vi "Begin Scripting Session.vi"(8 "error in":errorcluster, 10 "Undo Name":string, 11 "VI in":refnum<vi>) -> (0 "error out":errorcluster, 2 "Scripting Session":T1, 3 "VI out":refnum<vi>)   [LabVIEW 2020, in "Enclose in Structure.lvlib"]
uses:
  Enclose in Structure.lvlib
  Scripting Session.ctl
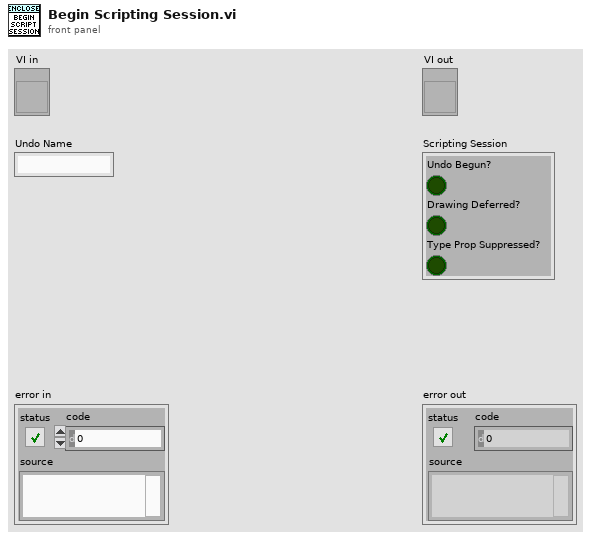
[diagram p1: front panel]
types:
  T1 = typedef "Enclose in Structure.lvlib/Scripting Session.ctl" = cluster{"Undo Begun?":bool, "Drawing Deferred?":bool, "Type Prop Suppressed?":bool}
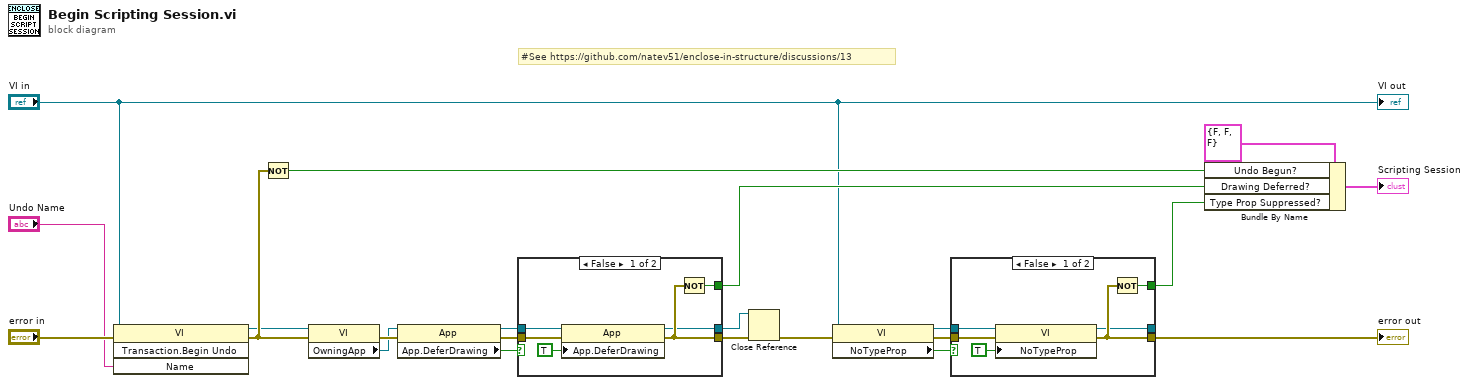
[diagram p0: block diagram]
diagram:
  # "#See https://github.com/natev51/enclose-in-structure/discussions/13"
  n1 = invoke class="VI" method="Transaction.Begin Undo"(reference="VI in", error in="error in", "Name"="Undo Name") -> (reference out=w4:refnum<vi>, error out=w22:errorcluster)  [unwired: 1 in, 2 out]
  n2 = Not(x=w22) -> (.not. x?=w2:bool)
  n3 = property class="VI"(reference=w4, error in=w22) -> (error out=w20:errorcluster, "OwningApp"=w19:refnum<vi>)  [unwired: 1 out]
  n4 = property class="App"(reference=w19, error in=w20) -> (reference out=w17:refnum<vi>, error out=w21:errorcluster, "App.DeferDrawing"=w13:bool)
  n5 = case shown="False" w13 {
    tunnel: w21 -> [w27 w29]
    tunnel: w17 -> [w26 w30]
    tunnel: [w28 w29] -> w16
    tunnel: [w25 w30] -> w15
    tunnel: [w23 _] -> w14
    frame False {
      n6 = property class="App"(reference=w26, error in=w27, "App.DeferDrawing"=TRUE ("Application:Defer Drawing")) -> (reference out=w25:refnum<vi>, error out=w28:errorcluster)
      n7 = Not(x=w28) -> (.not. x?=w23:bool)
    }
    frame True {
    }
  }
  n8 = Close Reference(reference=w15, error in (no error)=w16) -> (error out=w9:errorcluster)
  n9 = property class="VI"(reference="VI in", error in=w9) -> (reference out=w11:refnum<vi>, error out=w10:errorcluster, "NoTypeProp"=w12:bool)
  n10 = case shown="False" w12 {
    tunnel: w10 -> [w35 w37]
    tunnel: w11 -> [w34 w38]
    tunnel: [w36 w37] -> w6
    tunnel: [w33 w38] -> _
    tunnel: [w32 _] -> w8
    frame False {
      n11 = property class="VI"(reference=w34, error in=w35, "NoTypeProp"=TRUE ("Suppress Type Prop")) -> (reference out=w33:refnum<vi>, error out=w36:errorcluster)
      n12 = Not(x=w36) -> (.not. x?=w32:bool)
    }
    frame True {
    }
  }
  "error out" <- w6
  n13 = Bundle By Name(cluster=T1 {"Undo Begun?"=FALSE, "Drawing Deferred?"=FALSE, "Type Prop Suppressed?"=FALSE} ("Scripting Session"), "Undo Begun?"=w2, "Drawing Deferred?"=w14, "Type Prop Suppressed?"=w8) -> (→"Scripting Session":T1)
  "VI out" <- "VI in"
